vi "subFreqResp.vi"(9 "omega":dbl[](array[numeric]), 10 "a":cdb[](array[numeric]), 11 "b":cdb[](array[numeric])) -> (3 "Frequency Response":cdb[](array[numeric]))   [LabVIEW 2011]
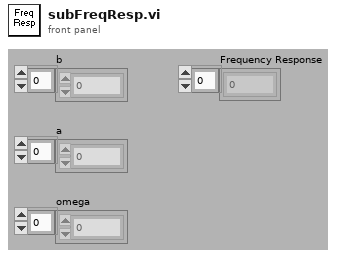
[diagram p1: front panel]
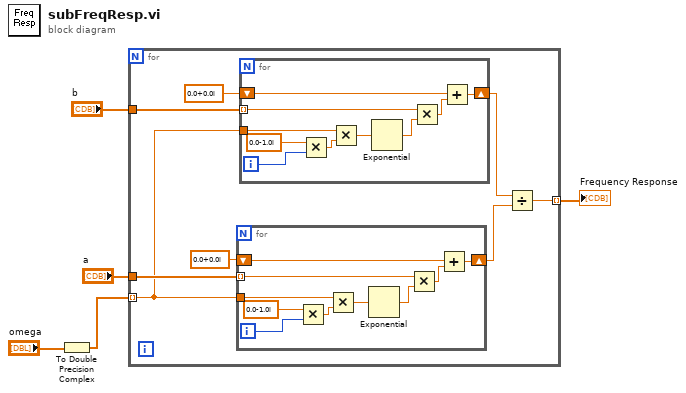
[diagram p0: block diagram]
diagram:
  n1 = To Double Precision Complex(1:"omega") -> (0:w3:cdb[])
  n2 = for {
    tunnel: "b" -> [w13]
    tunnel: [w6] -> w1 mode=indexing
    tunnel: w3 -> [w9] mode=indexing
    tunnel: "a" -> [w11]
    n3 = for {
      tunnel: w11 -> [w16] mode=indexing
      shift-right: [w17] -> w7
      shift-left: cdb 0.0+0.0i -> [w19]
      tunnel: w9 -> [w14]
      i -> [w23]
      n4 = Multiply(x=cdb 0.0-1.0i, y=w23) -> (x*y=w21:cdb)
      n5 = Multiply(x=w14, y=w21) -> (x*y=w20:cdb)
      n6 = Exponential(1:w20) -> (0:w15:cdb)
      n7 = Multiply(x=w16, y=w15) -> (x*y=w18:cdb)
      n8 = Add(x=w19, y=w18) -> (x+y=w17:cdb)
    }
    n9 = for {
      tunnel: w13 -> [w26] mode=indexing
      shift-right: [w27] -> w8
      shift-left: cdb 0.0+0.0i -> [w29]
      tunnel: w9 -> [w24]
      i -> [w33]
      n10 = Multiply(x=cdb 0.0-1.0i, y=w33) -> (x*y=w31:cdb)
      n11 = Multiply(x=w24, y=w31) -> (x*y=w30:cdb)
      n12 = Exponential(1:w30) -> (0:w25:cdb)
      n13 = Multiply(x=w26, y=w25) -> (x*y=w28:cdb)
      n14 = Add(x=w29, y=w28) -> (x+y=w27:cdb)
    }
    n15 = Divide(x=w8, y=w7) -> (x/y=w6:cdb)
  }
  "Frequency Response" <- w1
